vi "PathPlanner_ConstraintZone_Test.vi"(8 "error in (no error)":errorcluster) -> (0 "error out":errorcluster, 3 "All Passed":bool)   [LabVIEW 2019]
uses:
  <vilib>/Rock Robotics/WPI/ThirdParty/JAS_Junk/TrajLib/Trajectory_Library.lvlib
  <vilib>/Rock Robotics/WPI/ThirdParty/MJansen/PathPlanner/PathPlanner24.lvlib
panel:
  out "Passed 4":bool
  out "Passed 3":bool
  out "Passed 2":bool
  out "Passed 1":bool
  # "JSON Parse"
  # "Getters"
  # "Within Zone"
  # "Overlaps Range"
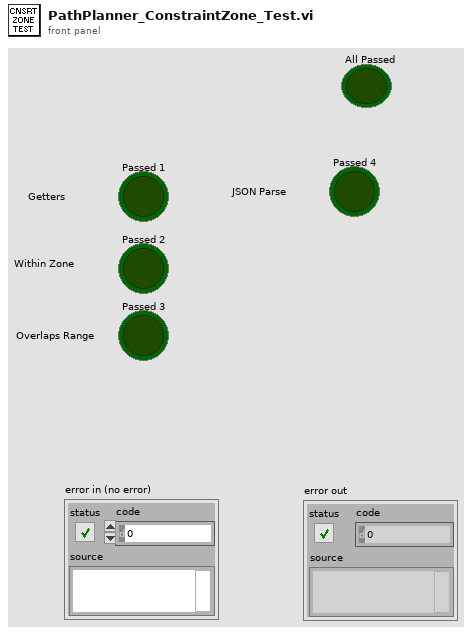
[diagram p1: front panel]
types:
  T1 = typedef "PathPlanner24.lvlib/PathPlannerPathConstraints.ctl" = cluster{"MaxVelocityMps;":dbl, "MaxAccelerationMpsSq;":dbl, "MaxAngularVelRadPsEc;":dbl, "MaxAngularAccRadPSecSq":dbl, "Exists":bool}
  T2 = typedef "PathPlanner24.lvlib/PathPlannerConstraintsZone.ctl" = cluster{"minWaypointPos":dbl, "maxWaypointPos":dbl, "Constraints":T1, "Present":bool}
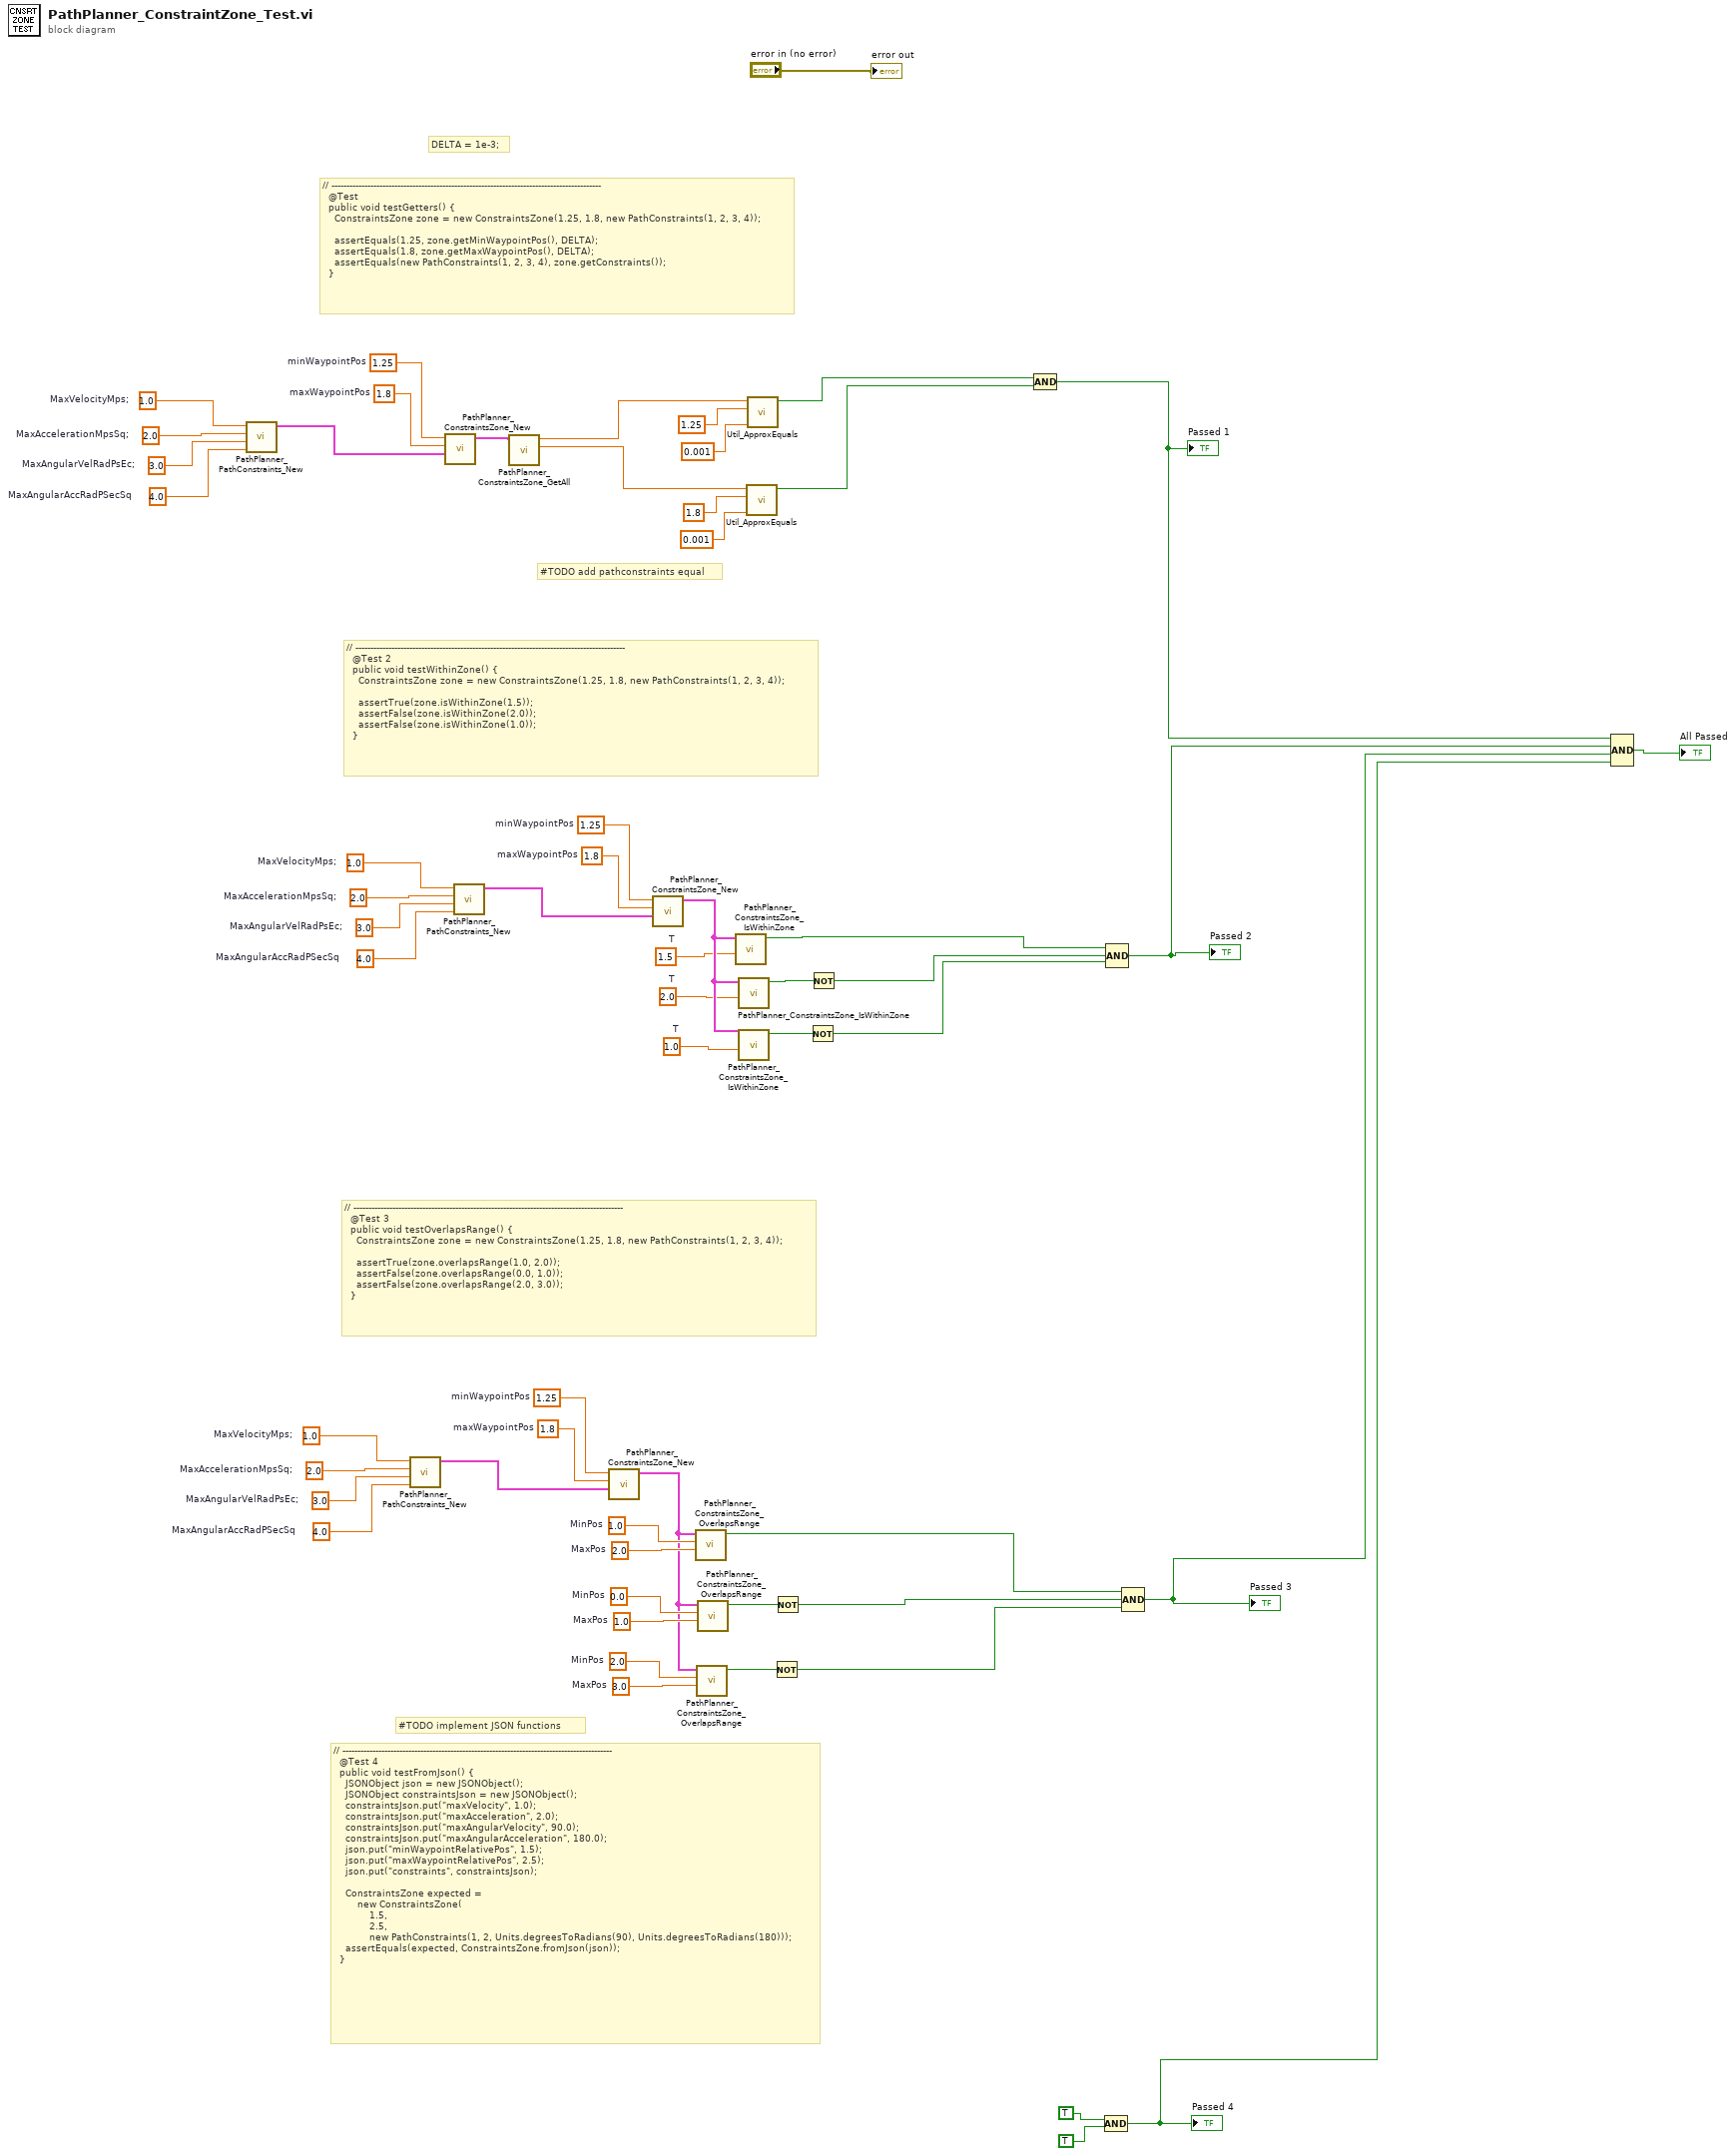
[diagram p0: block diagram]
diagram:
  w9 = 2.0  # MinPos
  w10 = 3.0  # MaxPos
  w11 = 0.0  # MinPos
  w12 = 1.0  # MaxPos
  w13 = 1.0  # MinPos
  w14 = 2.0  # MaxPos
  w16 = 1.8  # maxWaypointPos
  w17 = 1.25  # minWaypointPos
  w18 = 1.0  # MaxVelocityMps;
  w19 = 2.0  # MaxAccelerationMpsSq;
  w20 = 3.0  # MaxAngularVelRadPsEc;
  w21 = 4.0  # MaxAngularAccRadPSecSq
  w27 = 1.5  # T
  w28 = 2.0  # T
  w29 = 1.0  # T
  w32 = 1.8  # maxWaypointPos
  w33 = 1.25  # minWaypointPos
  w34 = 1.0  # MaxVelocityMps;
  w35 = 2.0  # MaxAccelerationMpsSq;
  w36 = 3.0  # MaxAngularVelRadPsEc;
  w37 = 4.0  # MaxAngularAccRadPSecSq
  w47 = 1.8  # maxWaypointPos
  w48 = 1.25  # minWaypointPos
  w49 = 1.0  # MaxVelocityMps;
  w50 = 2.0  # MaxAccelerationMpsSq;
  w51 = 3.0  # MaxAngularVelRadPsEc;
  w52 = 4.0  # MaxAngularAccRadPSecSq
  # "#TODO implement JSON functions"
  # "// ------------------------------------------------------------------------------------------\n  @Test 4\n  public void testFromJson() {\n    JSONObject json = new JSONObject();\n    JSONObject constraintsJson = new JSONObject();\n    constraintsJson.put(\"maxVelocity\", 1.0);\n    constraintsJson.put(\"maxAcceleration\", 2.0);\n    constraintsJson.put(\"maxAngularVelocity\", 90.0);\n    constraintsJson.put(\"maxAngularAcceleration\", 180.0);\n    json.put(\"minWaypointRelativePos\", 1.5);\n    json.put(\"maxWaypointRelativePos\", 2.5);\n    json.put(\"constraints\", constraintsJson);\n\n    ConstraintsZone expected =\n        new ConstraintsZone(\n            1.5,\n            2.5,\n            new PathConstraints(1, 2, Units.degreesToRadians(90), Units.degreesToRadians(180)));\n    assertEquals(expected, ConstraintsZone.fromJson(json));\n  }"
  # "// ------------------------------------------------------------------------------------------\n  @Test 3\n  public void testOverlapsRange() {\n    ConstraintsZone zone = new ConstraintsZone(1.25, 1.8, new PathConstraints(1, 2, 3, 4));\n\n    assertTrue(zone.overlapsRange(1.0, 2.0));\n    assertFalse(zone.overlapsRange(0.0, 1.0));\n    assertFalse(zone.overlapsRange(2.0, 3.0));\n  }"
  # "// ------------------------------------------------------------------------------------------\n  @Test 2\n  public void testWithinZone() {\n    ConstraintsZone zone = new ConstraintsZone(1.25, 1.8, new PathConstraints(1, 2, 3, 4));\n\n    assertTrue(zone.isWithinZone(1.5));\n    assertFalse(zone.isWithinZone(2.0));\n    assertFalse(zone.isWithinZone(1.0));\n  }"
  # "#TODO add pathconstraints equal"
  # "DELTA = 1e-3;"
  # "// ------------------------------------------------------------------------------------------\n  @Test\n  public void testGetters() {\n    ConstraintsZone zone = new ConstraintsZone(1.25, 1.8, new PathConstraints(1, 2, 3, 4));\n\n    assertEquals(1.25, zone.getMinWaypointPos(), DELTA);\n    assertEquals(1.8, zone.getMaxWaypointPos(), DELTA);\n    assertEquals(new PathConstraints(1, 2, 3, 4), zone.getConstraints());\n  }"
  n1 = call <vilib>:"PathPlanner_PathConstraints_New.vi"("MaxAngularAccRadPSecSq"=w52, "MaxAngularVelRadPsEc;"=w51, "MaxAccelerationMpsSq;"=w50, "MaxVelocityMps;"=w49) -> ("PathPlannerConstraints"=w46:T1)  [unwired: 7 in]
  n2 = call <vilib>:"PathPlanner_PathConstraints_New.vi"("MaxAngularAccRadPSecSq"=w21, "MaxAngularVelRadPsEc;"=w20, "MaxAccelerationMpsSq;"=w19, "MaxVelocityMps;"=w18) -> ("PathPlannerConstraints"=w15:T1)  [unwired: 7 in]
  n3 = call <vilib>:"PathPlanner_ConstraintsZone_New.vi"("Constraints"=w46, "maxWaypointPos"=w47, "minWaypointPos"=w48) -> ("ConstraintsZone"=w45:T2)  [unwired: 8 in]
  n4 = call <vilib>:"PathPlanner_PathConstraints_New.vi"("MaxAngularAccRadPSecSq"=w37, "MaxAngularVelRadPsEc;"=w36, "MaxAccelerationMpsSq;"=w35, "MaxVelocityMps;"=w34) -> ("PathPlannerConstraints"=w31:T1)  [unwired: 7 in]
  n5 = call <vilib>:"PathPlanner_ConstraintsZone_GetAll.vi"("ConstraintsZone"=w45) -> ("maxWaypointPos"=w39:dbl, "minWaypointPos"=w44:dbl)  [unwired: 8 in, 1 out]
  n6 = call <vilib>:"PathPlanner_ConstraintsZone_New.vi"("Constraints"=w15, "maxWaypointPos"=w16, "minWaypointPos"=w17) -> ("ConstraintsZone"=w6:T2)  [unwired: 8 in]
  n7 = call <vilib>:"PathPlanner_ConstraintsZone_New.vi"("Constraints"=w31, "maxWaypointPos"=w32, "minWaypointPos"=w33) -> ("ConstraintsZone"=w30:T2)  [unwired: 8 in]
  n8 = call <vilib>:"PathPlanner_ConstraintsZone_OverlapsRange.vi"("MaxPos"=w14, "MinPos"=w13, "ConstraintsZone"=w6) -> ("OverlapsRange"=w8:bool)  [unwired: 8 in]
  n9 = call <vilib>:"PathPlanner_ConstraintsZone_OverlapsRange.vi"("MaxPos"=w10, "MinPos"=w9, "ConstraintsZone"=w6) -> ("OverlapsRange"=w5:bool)  [unwired: 8 in]
  n10 = call <vilib>:"PathPlanner_ConstraintsZone_OverlapsRange.vi"("MaxPos"=w12, "MinPos"=w11, "ConstraintsZone"=w6) -> ("OverlapsRange"=w7:bool)  [unwired: 8 in]
  n11 = call <vilib>:"PathPlanner_ConstraintsZone_IsWithinZone.vi"("T"=w27, "ConstraintsZone"=w30) -> ("WithinZone"=w25:bool)  [unwired: 9 in]
  n12 = call <vilib>:"PathPlanner_ConstraintsZone_IsWithinZone.vi"("T"=w28, "ConstraintsZone"=w30) -> ("WithinZone"=w26:bool)  [unwired: 9 in]
  n13 = call <vilib>:"PathPlanner_ConstraintsZone_IsWithinZone.vi"("T"=w29, "ConstraintsZone"=w30) -> ("WithinZone"=w23:bool)  [unwired: 9 in]
  n14 = call <vilib>:"Util_ApproxEquals.vi"("Tolerance"=0.001, "Value 2"=1.8, "Value 1"=w39) -> ("ApproxEquals"=w38:bool)  [unwired: 8 in]
  n15 = call <vilib>:"Util_ApproxEquals.vi"("Tolerance"=0.001, "Value 2"=1.25, "Value 1"=w44) -> ("ApproxEquals"=w57:bool)  [unwired: 8 in]
  n16 = Not(x=w5) -> (.not. x?=w3:bool)
  n17 = Not(x=w7) -> (.not. x?=w4:bool)
  n18 = Not(x=w23) -> (.not. x?=w22:bool)
  n19 = Not(x=w26) -> (.not. x?=w24:bool)
  n20 = Compound Arithmetic op=AND(w57, w38) -> (w56:bool)
  "Passed 1" <- w56
  n21 = Compound Arithmetic op=AND(TRUE, TRUE) -> (w53:bool)
  "Passed 4" <- w53
  n22 = Compound Arithmetic op=AND(w25, w24, w22) -> (w55:bool)
  "Passed 2" <- w55
  n23 = Compound Arithmetic op=AND(w8, w4, w3) -> (w54:bool)
  "Passed 3" <- w54
  n24 = Compound Arithmetic op=AND(w56, w55, w54, w53) -> (→"All Passed":bool)
  "error out" <- "error in (no error)"
